vi "Teleop (2).vi"(10 "Match Info":T2={"Autonomous Elapsed Seconds"=0.0, "TeleOp Elapsed Seconds"=0.0, "Disabled Elapsed Seconds"=0.0, "Visited Autonomous"=FALSE, "Visited TeleOp"=FALSE, "Visited Disabled"=FALSE, "Autonomous Settings"={"Autonomous Style"=enum."Independent", "VI Refnum"=refnum}}, 11 "Call Context":T3) -> ()   [LabVIEW 2016]
doc: "This VI is called for each TeleOp packet received from the DS where the robot is not disabled. It is often used to read from the joysticks and update I/O or to update setpoints for timed control loops. It should complete and return within 20 milliseconds or it may miss DS packets."
uses:
  <vilib>/Rock Robotics/WPI/DriverStation/WPI_DriverStationDerivedRobotMode.ctl
  <vilib>/Rock Robotics/WPI/DriverStation/WPI_DriverStationMatch Info.ctl
  <vilib>/Rock Robotics/SystemInterfaces/AI/FPGA_AIGyroChannel.ctl
  <vilib>/Rock Robotics/Network Tables/NT Read Boolean.vi
  <vilib>/Rock Robotics/Network Tables/NT Read Number.vi
  <vilib>/Rock Robotics/WPI/Utilities/WPI_GetSetVariantRefNum.vi
  <vilib>/Rock Robotics/Network Tables/NT Write Boolean.vi
  <vilib>/Rock Robotics/Network Tables/NT Write Number.vi
  <vilib>/Rock Robotics/Network Tables/NT Write Boolean Array.vi
  <vilib>/Rock Robotics/Network Tables/NT Write Numeric Array.vi
  <vilib>/Rock Robotics/WPI/Solenoid/Deprecated/WPI_SolenoidSetBool.vi
  <vilib>/Rock Robotics/WPI/Ultrasonic/WPI_SonarMB1010AnalogRefNum Registry Get.vi
  <vilib>/Rock Robotics/WPI/Ultrasonic/WPI_SonarMB1010AnalogGetRange.vi
  PDP Currents Variable.vi
  <vilib>/Rock Robotics/WPI/Gyro/WPI_GyroAnalogOpen.vi
panel:
  out "gyro":dbl
  out "sonar distance (inches)":dbl
  out "Encoder Loop 2":string
  out "Encoder Loop":dbl
  out "gyro step two":dbl
  out "Encoder Rate":dbl
  out "Encoder State":string
  out "Encoder Direction":string
  out "Distance 2":dbl
  out "Angle 2":dbl
  out "Distance":dbl
  in  "Gain (VoltsPerDegree/Second)":dbl=0.007
  in  "Channel":T1
  in  "Reset Zero Position":bool
  in  "stop":bool
  out "Angle":dbl(knob) scale=0.0..360.0
  out "all currents (A) 2":dbl[](array[numeric])
  out "all currents (A)":dbl[](array[numeric])
  out "Enabled":bool
  out "Compressor Running":bool
  out "Sample Slider 0":dbl(slide) scale=0.0..5.0
  out "Sample Boolean 1":bool
  out "Sample Boolean 0":bool
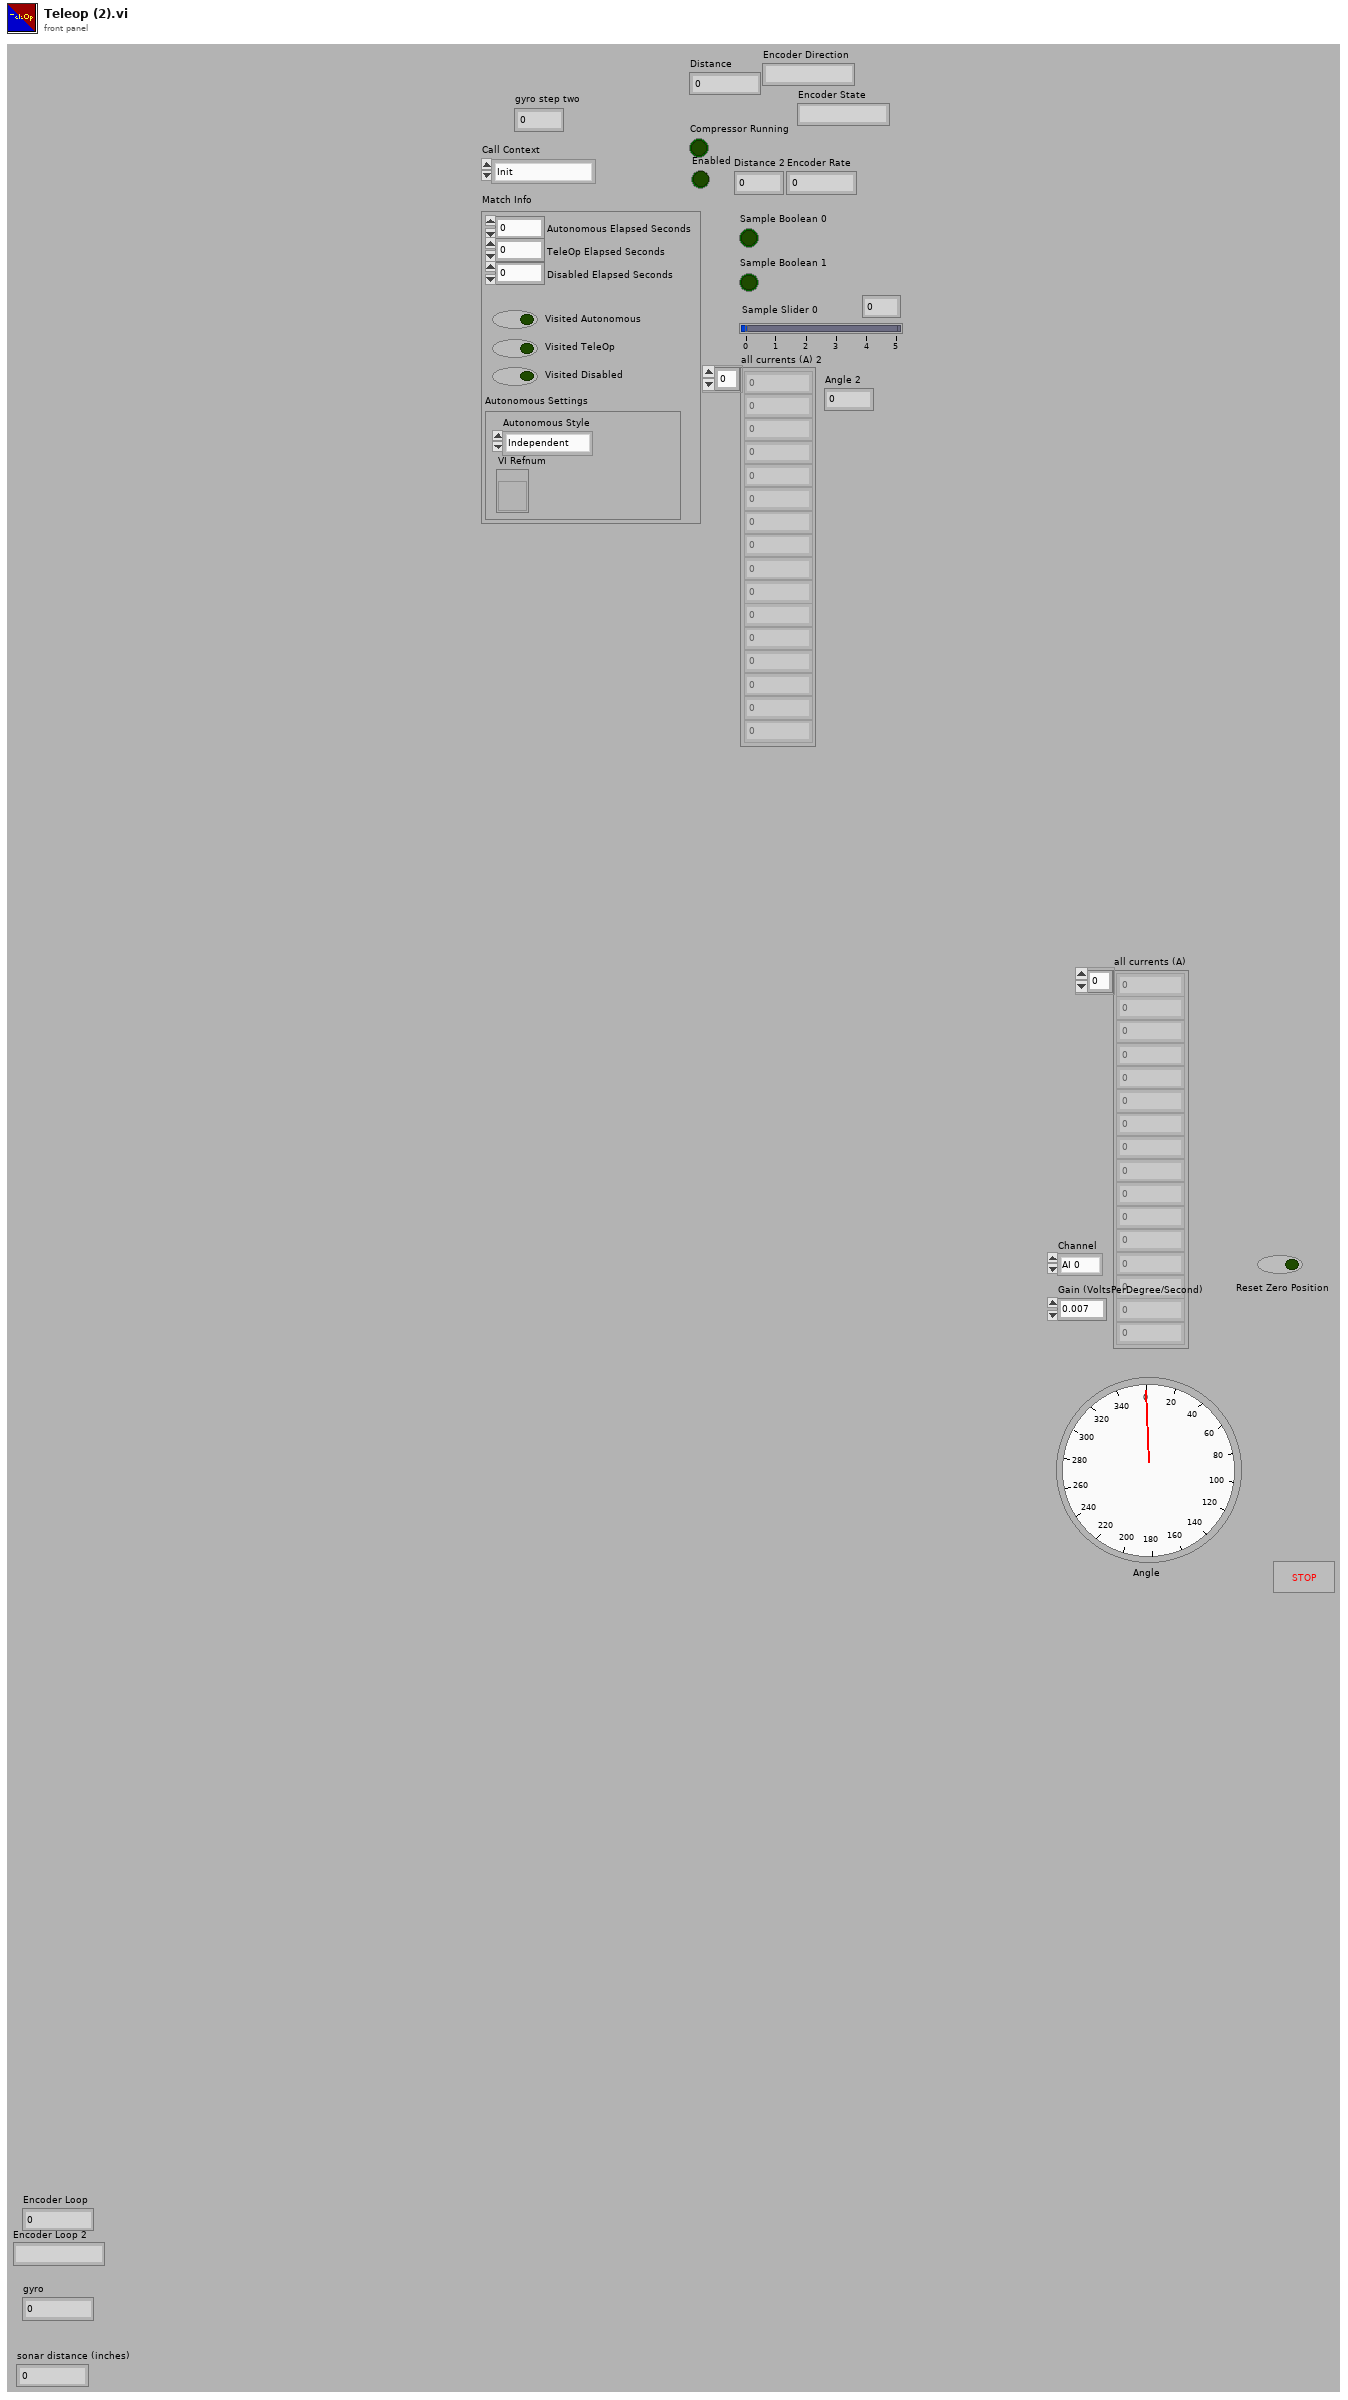
[diagram p1: front panel]
types:
  T1 = typedef "FPGA_AIGyroChannel.ctl" = enum8{"AI 0", "AI 1", "Invalid"}
  T2 = typedef "WPI_DriverStationMatch Info.ctl" = cluster{"Autonomous Elapsed Seconds":dbl, "TeleOp Elapsed Seconds":dbl, "Disabled Elapsed Seconds":dbl, "Visited Autonomous":bool, "Visited TeleOp":bool, "Visited Disabled":bool, "Autonomous Settings":cluster{"Autonomous Style":enum16{"Iterative", "Independent"}, "VI Refnum":refnum<vi>}}
  T3 = typedef "WPI_DriverStationDerivedRobotMode.ctl" = enum16{"Init", "Execute", "Stop"}
  T4 = typedef "WPI_JoystickDevRef.ctl" = cluster{"Device":T5}
  T5 = typedef "WPI_JoystickDeviceEnum.ctl" = enum16{"USB 0", "USB 1", "USB 2", "USB 3", "USB 4", "USB 5"}
  T6 = typedef "WPI_CompressorDevRef.ctl" = cluster{"DevStatus":errorcluster, "Pneumatics Control Module":u8}
  T7 = typedef "WPI_SonarMB1010AnalogDeviceRef.ctl" = cluster{"AIDeviceRef":T8, "Scaling factor (V/in)":dbl, "Average Bits":u8}
  T8 = typedef "WPI_AnalogChannelDevRef.ctl" = cluster{"DevStatus":errorcluster, "Analog Channel":T9}
  T9 = typedef "FPGA_AIChannel.ctl" = enum8{"AI 0", "AI 1", "AI 2", "AI 3", "AI MXP 0", "AI MXP 1", "AI MXP 2", "AI MXP 3", "Invalid"}
  T10 = typedef "WPI_SolenoidDevRef.ctl" = cluster{"DevStatus":errorcluster, "Pneumatics Control Module":u8, "Forward Solenoid Channel":T11, "Reverse Solenoid Channel":T11}
  T11 = typedef "WPI_SolenoidChannel.ctl" = enum8{"Solenoid 0", "Solenoid 1", "Solenoid 2", "Solenoid 3", "Solenoid 4", "Solenoid 5", "Solenoid 6", "Solenoid 7", "Invalid"}
  T12 = typedef "WPI_SwitchDevRef.ctl" = cluster{"DevStatus":errorcluster, "DIO Channel":T13, "CntIndex":T14, "Normally Closed":bool}
  T13 = typedef "FPGA_DIOChannel.ctl" = enum8{"DIO 0", "DIO 1", "DIO 2", "DIO 3", "DIO 4", "DIO 5", "DIO 6", "DIO 7", "DIO 8", "DIO 9", "DIO MXP 0", "DIO MXP 1", "DIO MXP 2", "DIO MXP 3", "DIO MXP 4", "DIO MXP 5", "DIO MXP 6", "DIO MXP 7", "DIO MXP 8", "DIO MXP 9", "DIO MXP 10", "DIO MXP 11", "DIO MXP 12", "DIO MXP 13", "DIO MXP 14", "DIO MXP 15", "SPI Port CS1", "SPI Port CS2", "SPI Port CS3", "SPI Port MISO", "SPI Port MOSI", "Invalid"}
  T14 = typedef "FPGA_CounterCtrSystemIndex.ctl" = enum8{"Ctr 0", "Ctr 1", "Ctr 2", "Ctr 3", "Ctr 4", "Ctr 5", "Ctr 6", "Ctr 7", "Invalid"}
  T15 = typedef "WPI_RobotDriveDevRef.ctl" = cluster{"DevStatus":errorcluster, "Motors[]":T16[], "Square Inputs":bool, "Max Output":dbl}
  T16 = typedef "WPI_MotorControlDeviceRef.ctl" = cluster{"DeviceStatus":errorcluster, "Type":T17, "PWM":cluster{"PWM Channel":T18, "DeadBand":T19}, "CAN":cluster{"Device Number":u8, "SetOutput VI Ref":variant, "GetOutput VI Ref":variant, "Enable VI Ref":variant, "Disable VI Ref":variant, "Data":variant}, "Invert":bool}
  T17 = typedef "WPI_MotorControlType.ctl" = enum16{"PWM", "CAN"}
  T18 = typedef "FPGA_DIOPWMChannel.ctl" = enum8{"PWM 0", "PWM 1", "PWM 2", "PWM 3", "PWM 4", "PWM 5", "PWM 6", "PWM 7", "PWM 8", "PWM 9", "PWM MXP 0", "PWM MXP 1", "PWM MXP 2", "PWM MXP 3", "PWM MXP 4", "PWM MXP 5", "PWM MXP 6", "PWM MXP 7", "PWM MXP 8", "PWM MXP 9", "Invalid"}
  T19 = typedef "WPI_PWMDeadband.ctl" = cluster{"Name":string, "maxPositivePwm":i32, "minPositivePwm":i32, "centerPwm":i32, "maxNegativePwm":i32, "minNegativePwm":i32, "angularRange":u16}
  T20 = typedef "WPI_GyroDevRef.ctl" = cluster{"DevStatus":errorcluster, "Analog Channel":T9, "Offset":dbl, "Gain (VoltsPerDegree/Second)":dbl, "Gyro Type":enum16{"Analog", "XRS450"}, "Handle":i32, "SPI Bus":T21, "Device Found":bool, "Sample Rate":dbl, "Calibrate On Open":bool}
  T21 = typedef "spi_bus.ctl" = enum16{"SPI On-Board, CS0", "SPI On-Board, CS1", "SPI On-Board, CS2", "SPI On-Board, CS3", "SPI MXP", "Invalid"}
  T22 = typedef "WPI_EncoderDevRef.ctl" = cluster{"DevStatus":errorcluster, "EncoderIndex":T23, "CounterIndex":T14, "DistancePerCount":dbl, "Decoding Type":T24}
  T23 = typedef "FPGA_EncoderIdx.ctl" = enum8{"Enc 0", "Enc 1", "Enc 2", "Enc 3", "Enc 4", "Enc 5", "Enc 6", "Enc 7", "Invalid"}
  T24 = typedef "WPI_EncoderType.ctl" = enum16{"1x", "2x", "4x"}
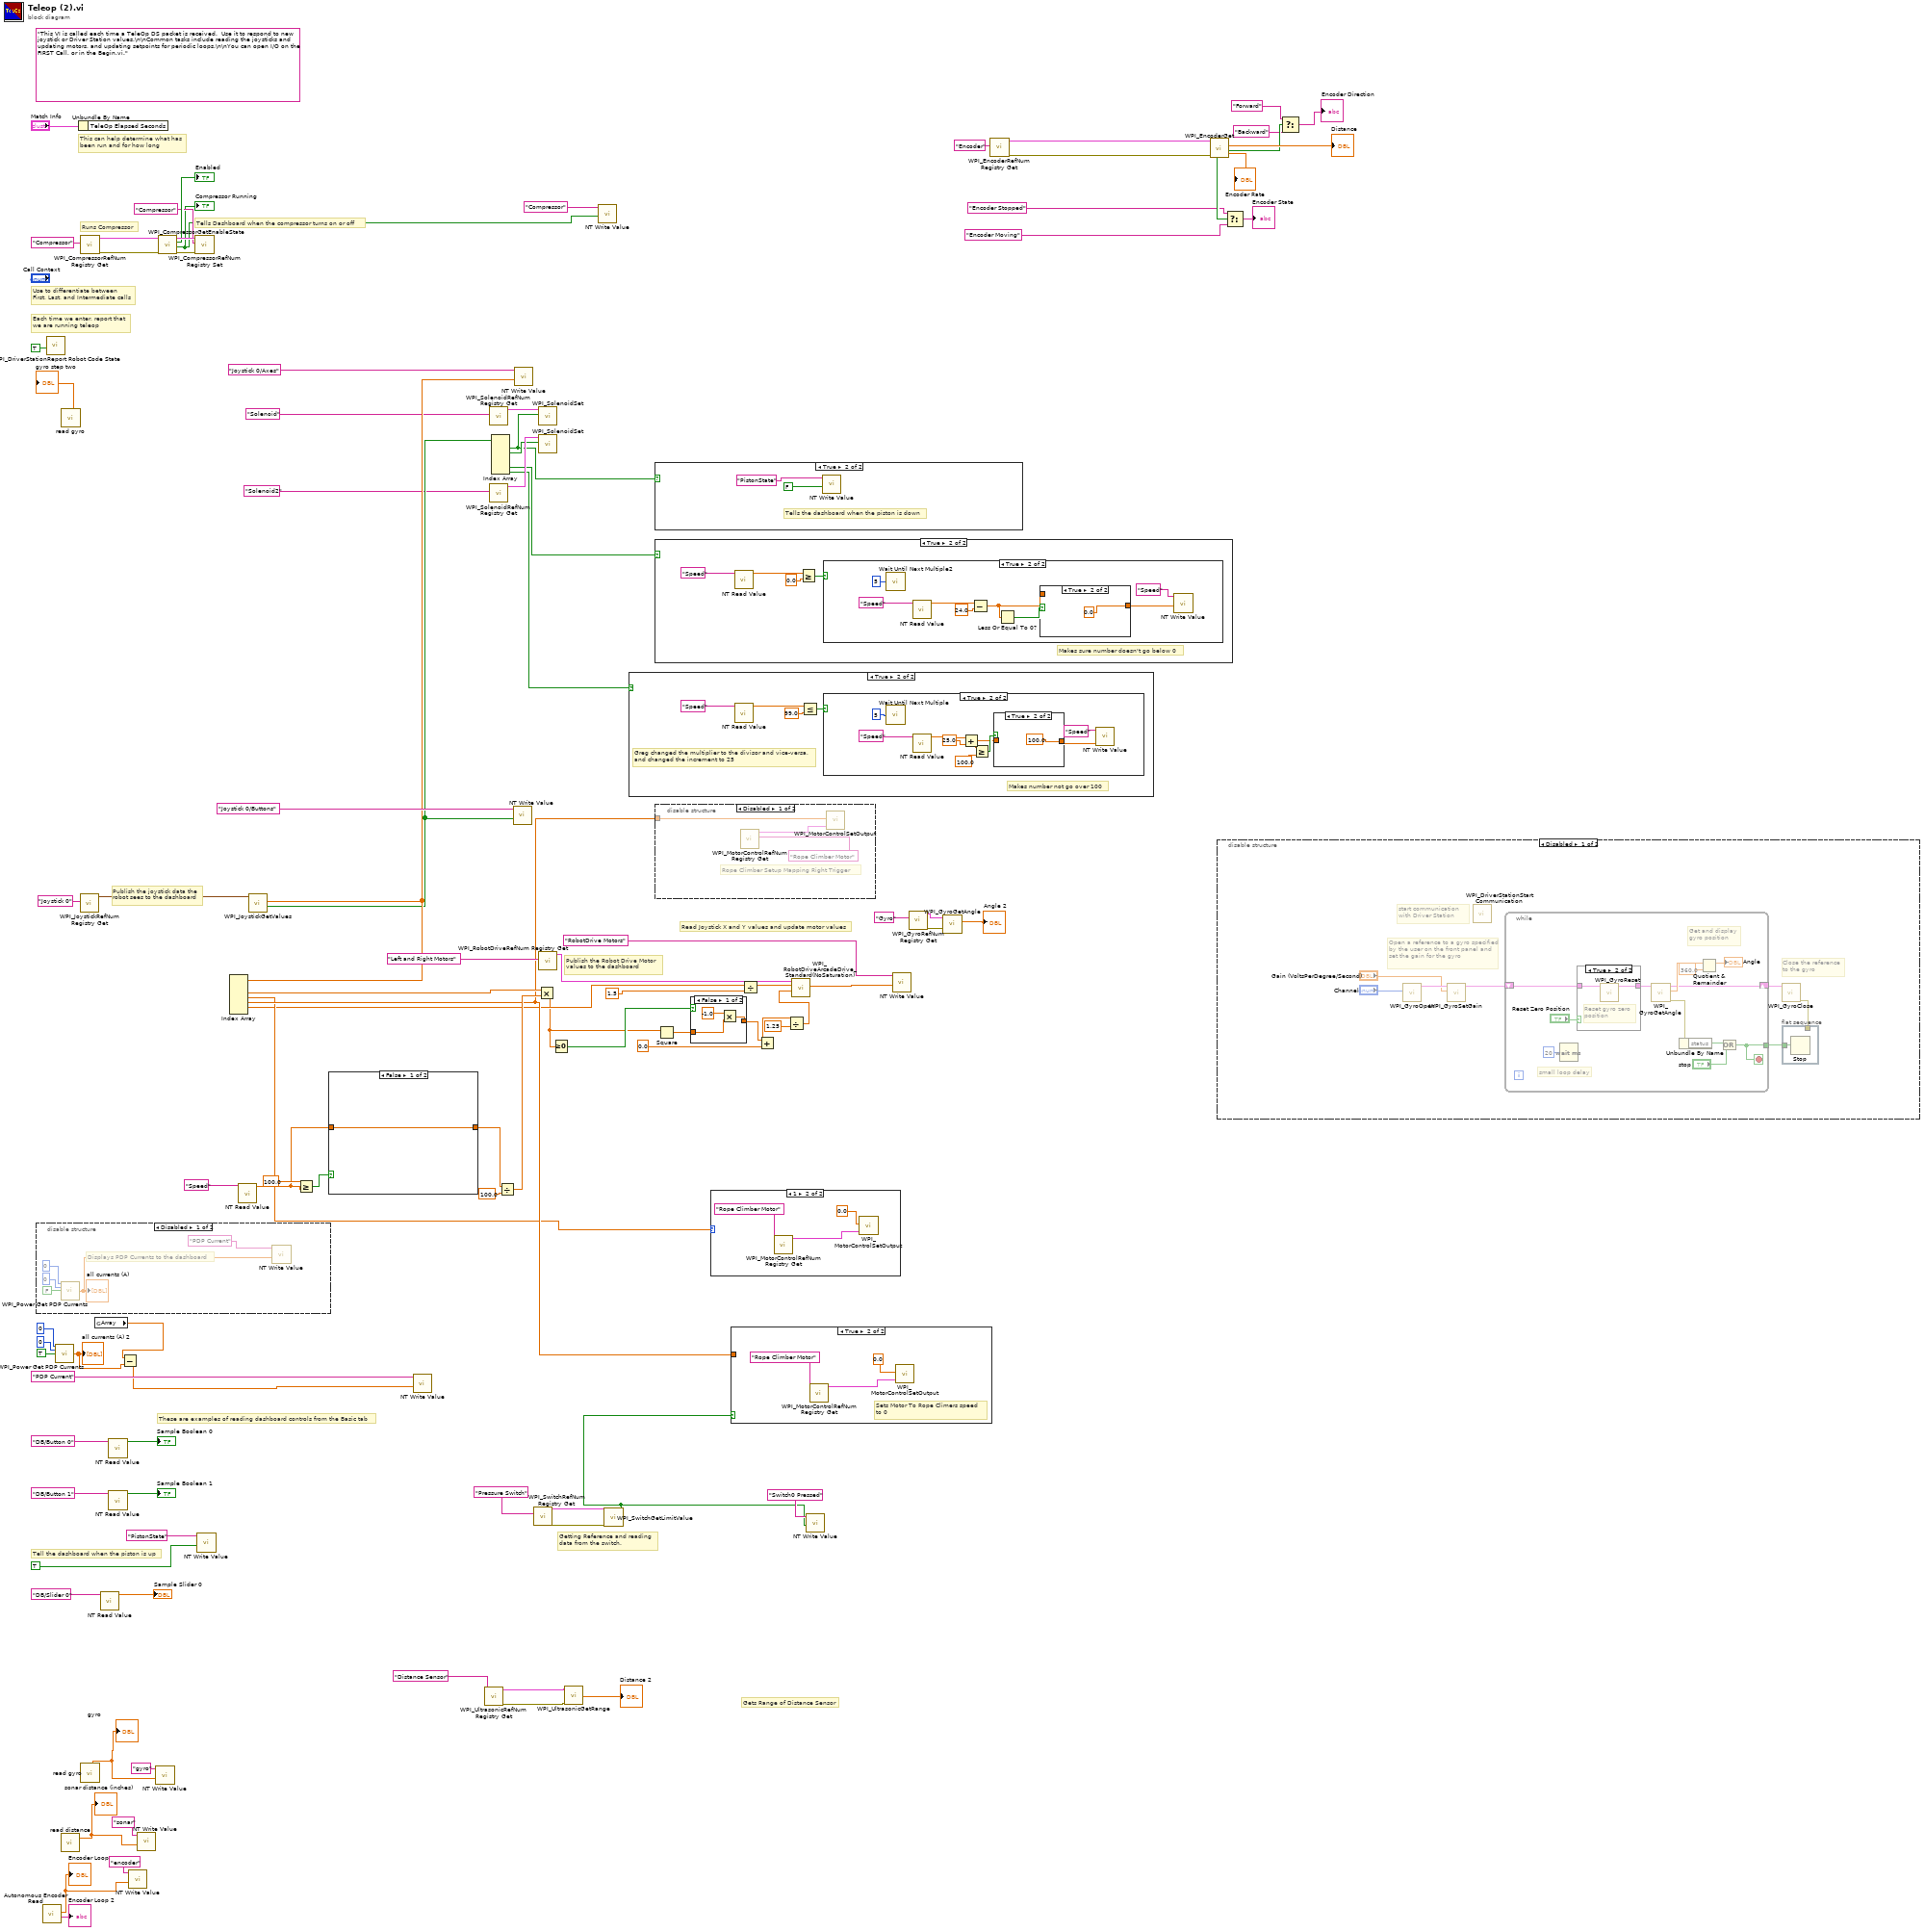
[diagram p0: block diagram]
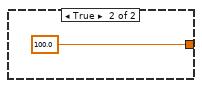
[diagram p3: hidden frame]
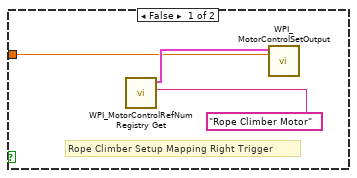
[diagram p8: hidden frame]
diagram:
  (unwired) "This VI is called each time a TeleOp DS packet is received.  Use it to respond to new joystick or Driver Station values.\n\nCommon tasks include reading the joysticks and updating motors, and updating setpoints for periodic loops.\n\nYou can open I/O on the FIRST Call, or in the Begin.vi."
  # "Gets Range of Distance Sensor"
  # "Getting Reference and reading \ndata from the switch."
  # "Tell the dashboard when the piston is up"
  # "Publish the joystick data the\nrobot sees to the dashboard"
  # "Publish the Robot Drive Motor\nvalues to the dashboard"
  # "Read Joystick X and Y values and update motor values"
  # "Tells Dashboard when the compressor turns on or off"
  # "Runs Compressor"
  # "These are examples of reading dashboard controls from the Basic tab"
  # "Each time we enter, report that\nwe are running teleop"
  # "Use to differentiate between\nFirst, Last, and Intermediate calls"
  # "This can help determine what has\nbeen run and for how long"
  n1 = disable-structure shown="Disabled" {
    frame Disabled {
      # "Displays PDP Currents to the dashboard"
      n2 = call <vilib>:"WPI_Power Get PDP Currents.vi"("Power Distribution Panel (0)"=u8 0, "PDP Channel"=0, "Tare Currents?"=FALSE) -> ("all currents (A)"=w102:dbl[])  [unwired: 10 in, 2 out]
      "all currents (A)" <- w102
      n3 = call-poly <vilib>:"NT Write Value.vi"("Numeric Array"=w102, "Name"="PDP Current") -> ()  [unwired: 9 in, 1 out]
    }
    frame Enabled {
    }
  }
  n4 = call "Autonomous Encoder Read.vi"() -> ("Encoder Direction"=→"Encoder Loop 2":string, "Encoder Distance"=w2:dbl)  [unwired: 9 in, 1 out]
  "Encoder Loop" <- w2
  n5 = call <vilib>:"WPI_DriverStationReport Robot Code State.vi"("TeleOp"=TRUE ("Autonomous")) -> ()  [unwired: 10 in, 1 out]
  n6 = call <vilib>:"WPI_Power Get PDP Currents.vi"("Power Distribution Panel (0)"=u8 0, "PDP Channel"=0, "Tare Currents?"=TRUE) -> ("all currents (A)"=w54:dbl[])  [unwired: 10 in, 2 out]
  "all currents (A) 2" <- w54
  n7 = call "read distance.vi"() -> ("Distance 2"=w5:dbl)  [unwired: 10 in, 1 out]
  "sonar distance (inches)" <- w5
  n8 = call "read gyro.vi"() -> ("Angle 2"=→"gyro step two":dbl)  [unwired: 10 in, 1 out]
  n9 = Unbundle By Name("Match Info") -> ()  [unwired: 1 out]
  n10 = call <vilib>:"WPI_JoystickRefNum Registry Get.vi"("refnum name"="Joystick 0") -> ("JoystickDevRef"=w79:T4)  [unwired: 1 in, 9 out]
  n11 = call <vilib>:"WPI_CompressorRefNum Registry Get.vi"("refnum name"="Compressor") -> ("error out"=w89:errorcluster, "CompressorDevRef"=w91:T6)  [unwired: 9 in]
  n12 = call "read gyro.vi"() -> ("Angle 2"=w7:dbl)  [unwired: 10 in, 1 out]
  "gyro" <- w7
  n13 = global read "PDP Currents Variable.vi" "Array"() -> (w52:dbl[])
  n14 = call-poly <vilib>:"NT Read Value.vi"("Name"="DB/Slider 0" ("refnum name")) -> ("Numeric"=→"Sample Slider 0":dbl)  [unwired: 9 in, 1 out]
  n15 = call-poly <vilib>:"NT Read Value.vi"("Name"="DB/Button 0" ("refnum name")) -> ("Boolean"=→"Sample Boolean 0":bool)  [unwired: 9 in, 1 out]
  n16 = call-poly <vilib>:"NT Read Value.vi"("Name"="DB/Button 1" ("refnum name")) -> ("Boolean"=→"Sample Boolean 1":bool)  [unwired: 9 in, 1 out]
  n17 = Subtract(x=w52, y=w54) -> (x-y=w53:dbl[])
  n18 = call-poly <vilib>:"NT Write Value.vi"("Numeric"=w2, "Name"="encoder") -> ()  [unwired: 9 in, 1 out]
  n19 = call-poly <vilib>:"NT Write Value.vi"("Numeric"=w5, "Name"="sonar") -> ()  [unwired: 9 in, 1 out]
  n20 = call-poly <vilib>:"NT Write Value.vi"("Numeric"=w7, "Name"="gyro") -> ()  [unwired: 9 in, 1 out]
  n21 = call <vilib>:"WPI_CompressorGetEnableState.vi"("error in (no error)"=w89, "CompressorDevRef"=w91) -> ("error out"=w88:errorcluster, "Compressor Running"=w83:bool, "Enabled"=→"Enabled":bool, "CompressorDevRef"=w90:T6)  [unwired: 6 in]
  "Compressor Running" <- w83
  n22 = call <vilib>:"WPI_CompressorRefNum Registry Set.vi"("error in (no error)"=w88, "refnum name"="Compressor", "CompressorDevRef"=w90) -> ()  [unwired: 7 in, 2 out]
  n23 = call-poly <vilib>:"NT Write Value.vi"("Boolean"=TRUE, "Name"="PistonState") -> ()  [unwired: 9 in, 1 out]
  n24 = call-poly <vilib>:"NT Read Value.vi"("Name"="Speed") -> ("Numeric"=w16:dbl)  [unwired: 9 in, 1 out]
  n25 = call <vilib>:"WPI_JoystickGetValues.vi"("JoystickDevRef"=w79) -> ("Buttons"=w73:bool[], "Axes"=w76:dbl[])  [unwired: 6 in, 3 out]
  n26 = Index Array(array=w76) -> (element #2=w64:dbl, element #3=w45:dbl, element #4=w46:dbl, element #5=w20:dbl)  [unwired: 6 in, 2 out]
  n27 = Greater Or Equal?(x=100.0, y=w16) -> (x >= y?=w18:bool)
  n28 = case shown="False" w18 {
    tunnel: [w105 100.0 ("Numeric")] -> w17
    tunnel: w16 -> [w105 _]
    frame False {
    }
    frame True {
    }
  }
  n29 = call-poly <vilib>:"NT Write Value.vi"("Numeric Array"=w53, "Name"="PDP Current") -> ()  [unwired: 9 in, 1 out]
  n30 = call-poly <vilib>:"WPI_UltrasonicRefNum Registry Get.vi"("refnum name"="Distance Sensor") -> ("error out"=w31:errorcluster, "SonarMB1010AnalogDevRef"=w33:T7)  [unwired: 9 in]
  n31 = call <vilib>:"WPI_SolenoidRefNum Registry Get.vi"("refnum name"="Solenoid") -> ("SolenoidDevRef"=w69:T10)  [unwired: 9 in, 1 out]
  n32 = call <vilib>:"WPI_SolenoidRefNum Registry Get.vi"("refnum name"="Solenoid2") -> ("SolenoidDevRef"=w71:T10)  [unwired: 9 in, 1 out]
  n33 = Index Array(array=w73) -> (element #1=w67:bool, element #2=w68:bool, element #5=w59:bool, element #6=w60:bool)  [unwired: 6 in, 2 out]
  n34 = Divide(x=w17, y=100.0 ("x")) -> (x/y=w61:dbl)
  n35 = call-poly <vilib>:"NT Write Value.vi"("Boolean Array"=w73, "Name"="Joystick 0/Buttons") -> ()  [unwired: 9 in, 1 out]
  n36 = call-poly <vilib>:"NT Write Value.vi"("Numeric Array"=w76, "Name"="Joystick 0/Axes") -> ()  [unwired: 9 in, 1 out]
  n37 = call <vilib>:"WPI_SwitchRefNum Registry Get.vi"("refnum name"="Pressure Switch") -> ("error out"=w49:errorcluster, "SwitchDevRef"=w50:T12)  [unwired: 9 in]
  n38 = Multiply(x=w64, y=w61) -> (x*y=w10:dbl)
  n39 = call-poly <vilib>:"WPI_SolenoidSet.vi"("Value"=w67, "SolenoidDevRef"=w69) -> ()  [unwired: 8 in, 2 out]
  n40 = call-poly <vilib>:"WPI_SolenoidSet.vi"("Value"=w68, "SolenoidDevRef"=w71) -> ()  [unwired: 8 in, 2 out]
  n41 = call <vilib>:"WPI_RobotDriveRefNum Registry Get.vi"("refnum name"="Left and Right Motors") -> ("RobotDriveDevRef"=w81:T15)  [unwired: 1 in, 9 out]
  n42 = Greater Or Equal To 0?(x=w10) -> (x >= 0?=w11:bool)
  n43 = call-poly <vilib>:"WPI_UltrasonicGetRange.vi"("error in"=w31, "SonarMB1010AnalogDevRef"=w33) -> ("Distance"=→"Distance 2":dbl)  [unwired: 7 in, 2 out]
  n44 = call-poly <vilib>:"NT Write Value.vi"("Boolean"=w83, "Name"="Compressor") -> ()  [unwired: 9 in, 1 out]
  n45 = call <vilib>:"WPI_SwitchGetLimitValue.vi"("error in (no error)"=w49, "SwitchDevRef"=w50) -> ("Switch Pressed"=w47:bool)  [unwired: 7 in, 2 out]
  n46 = case shown="True" w60 {
    frame False {
    }
    frame True {
      # "Makes number not go over 100"
      # "Greg changed the multiplier to the divisor and vice-versa,\nand changed the increment to 25"
      n47 = call-poly <vilib>:"NT Read Value.vi"("Name"="Speed") -> ("Numeric"=w108:dbl)  [unwired: 9 in, 1 out]
      n48 = Less Or Equal?(x=w108, y=99.0) -> (x <= y?=w109:bool)
      n49 = case shown="True" w109 {
        frame False {
        }
        frame True {
          n50 = call "Wait Until Next Multiple"("Count(mSec)"=u32 5) -> ()  [unwired: 1 out]
          n51 = call-poly <vilib>:"NT Read Value.vi"("Name"="Speed") -> ("Numeric"=w116:dbl)  [unwired: 9 in, 1 out]
          n52 = Add(x=w116, y=25.0) -> (x+y=w111:dbl)
          n53 = Greater Or Equal?(x=w111, y=100.0) -> (x >= y?=w113:bool)
          n54 = case shown="True" w113 {
            tunnel: [w120 100.0 ("Numeric")] -> w114
            tunnel: w111 -> [w120 _]
            frame False {
            }
            frame True {
            }
          }
          n55 = call-poly <vilib>:"NT Write Value.vi"("Numeric"=w114, "Name"="Speed") -> ()  [unwired: 9 in, 1 out]
        }
      }
    }
  }
  n56 = case shown="True" w67 {
    frame False {
    }
    frame True {
      # "Tells the dashboard when the piston is down"
      n57 = call-poly <vilib>:"NT Write Value.vi"("Boolean"=FALSE, "Name"="PistonState") -> ()  [unwired: 9 in, 1 out]
    }
  }
  n58 = case shown="True" w59 {
    frame False {
    }
    frame True {
      # "Makes sure number doesn't go below 0"
      n59 = call-poly <vilib>:"NT Read Value.vi"("Name"="Speed") -> ("Numeric"=w126:dbl)  [unwired: 9 in, 1 out]
      n60 = Greater Or Equal?(x=w126, y=0.0) -> (x >= y?=w124:bool)
      n61 = case shown="True" w124 {
        frame False {
        }
        frame True {
          n62 = call "Wait Until Next Multiple2"("Count(mSec)"=u32 5) -> ()  [unwired: 1 out]
          n63 = call-poly <vilib>:"NT Read Value.vi"("Name"="Speed") -> ("Numeric"=w134:dbl)  [unwired: 9 in, 1 out]
          n64 = Subtract(x=w134, y=24.0) -> (x-y=w128:dbl)
          n65 = Less Or Equal To 0?(x=w128) -> (x <= 0?=w130:bool)
          n66 = case shown="True" w130 {
            tunnel: [w136 0.0 ("Numeric")] -> w129
            tunnel: w128 -> [w136 _]
            frame False {
            }
            frame True {
            }
          }
          n67 = call-poly <vilib>:"NT Write Value.vi"("Numeric"=w129, "Name"="Speed") -> ()  [unwired: 9 in, 1 out]
        }
      }
    }
  }
  n68 = disable-structure shown="Disabled" {
    disable-tunnel: w46 -> [w138 _]
    frame Disabled {
      # "Rope Climber Setup Mapping Right Trigger"
      n69 = call <vilib>:"WPI_MotorControlRefNum Registry Get.vi"("refnum name"="Rope Climber Motor") -> ("MotorControlDevRef"=w139:T16)  [unwired: 9 in, 1 out]
      n70 = call <vilib>:"WPI_MotorControlSetOutput.vi"("Output"=w138, "MotorControlDevRef"=w139) -> ()  [unwired: 7 in, 3 out]
    }
    frame Enabled {
    }
  }
  n71 = Square(x=w10) -> (x^2=w9:dbl)
  n72 = case shown="False" w11 {
    tunnel: w9 -> [w143 w144]
    tunnel: [w141 w144] -> w8
    frame False {
      n73 = Multiply(x=-1.0, y=w143) -> (x*y=w141:dbl)
    }
    frame True {
    }
  }
  n74 = case shown="1" w45 {
    frame 0, Default {
    }
    frame 1 {
      n75 = call <vilib>:"WPI_MotorControlRefNum Registry Get.vi"("refnum name"="Rope Climber Motor") -> ("MotorControlDevRef"=w147:T16)  [unwired: 9 in, 1 out]
      n76 = call <vilib>:"WPI_MotorControlSetOutput.vi"("Output"=0.0 ("Motor Output"), "MotorControlDevRef"=w147) -> ()  [unwired: 7 in, 3 out]
    }
  }
  n77 = case shown="True" w47 {
    tunnel: w46 -> [w148 _]
    frame False {
      # "Rope Climber Setup Mapping Right Trigger"
      n78 = call <vilib>:"WPI_MotorControlRefNum Registry Get.vi"("refnum name"="Rope Climber Motor") -> ("MotorControlDevRef"=w149:T16)  [unwired: 9 in, 1 out]
      n79 = call <vilib>:"WPI_MotorControlSetOutput.vi"("Output"=w148, "MotorControlDevRef"=w149) -> ()  [unwired: 7 in, 3 out]
    }
    frame True {
      # "Sets Motor To Rope Climers speed \nto 0"
      n80 = call <vilib>:"WPI_MotorControlRefNum Registry Get.vi"("refnum name"="Rope Climber Motor") -> ("MotorControlDevRef"=w153:T16)  [unwired: 9 in, 1 out]
      n81 = call <vilib>:"WPI_MotorControlSetOutput.vi"("Output"=0.0 ("Motor Output"), "MotorControlDevRef"=w153) -> ()  [unwired: 7 in, 3 out]
    }
  }
  n82 = Divide(x=w20, y=1.5) -> (x/y=w43:dbl)
  n83 = Add(x=w8, y=0.0) -> (x+y=w13:dbl)
  n84 = Divide(x=w13, y=1.25) -> (x/y=w12:dbl)
  n85 = call <vilib>:"WPI_RobotDriveArcadeDrive_Standard(NoSaturation).vi"("Y axis value"=w12, "X axis value"=w43, "RobotDriveDevRef"=w81) -> ("Motor Values"=w75:dbl[])  [unwired: 1 in, 7 out]
  n86 = call-poly <vilib>:"NT Write Value.vi"("Boolean"=w47, "Name"="Switch0 Pressed") -> ()  [unwired: 9 in, 1 out]
  n87 = call-poly <vilib>:"NT Write Value.vi"("Numeric Array"=w75, "Name"="RobotDrive Motors") -> ()  [unwired: 9 in, 1 out]
  n88 = call <vilib>:"WPI_GyroRefNum Registry Get.vi"("refnum name"="Gyro") -> ("error out"=w35:errorcluster, "GyroDevRef"=w36:T20)  [unwired: 9 in]
  n89 = call <vilib>:"WPI_GyroGetAngle.vi"("error in"=w35, "GyroDevRef"=w36) -> ("Angle"=→"Angle 2":dbl)  [unwired: 5 in, 4 out]
  n90 = call <vilib>:"WPI_EncoderRefNum Registry Get.vi"("refnum name"="Encoder") -> ("error out"=w40:errorcluster, "EncoderDevRef"=w41:T22)  [unwired: 9 in]
  n91 = call <vilib>:"WPI_EncoderGet.vi"("error in (no error)"=w40, "EncoderDevRef"=w41) -> ("Direction"=w30:bool, "Distance"=→"Distance":dbl, "Rate"=→"Encoder Rate":dbl, "Stopped"=w26:bool)  [unwired: 4 in, 2 out]
  n92 = disable-structure shown="Disabled" {
    frame Disabled {
      # "start communication with Driver Station"
      # "Close the reference\nto the gyro"
      # "Open a reference to a gyro specified by the user on the front panel and set the gain for the gyro"
      n93 = call-poly <vilib>:"WPI_GyroOpen.vi"("Analog Channel"="Channel") -> ("GyroDevRef"=w159:T20)  [unwired: 8 in, 2 out]
      n94 = call <vilib>:"WPI_GyroSetGain.vi"("Gain (VoltsPerDegree/Second)"="Gain (VoltsPerDegree/Second)", "GyroDevRef"=w159) -> ("GyroDevRef"=w158:T20)  [unwired: 1 in, 8 out]
      n95 = call <vilib>:"WPI_DriverStationStart Communication.vi"() -> ()  [unwired: 2 in, 10 out]
      n96 = while {
        shift-right: [w169] -> w160
        shift-left: w158 -> [w172]
        tunnel: [w167] -> w155
        stop <- w167 stop-if-true
        # "small loop delay"
        # "Get and display\ngyro position"
        n97 = Wait (ms)(milliseconds to wait=u32 20) -> ()  [unwired: 1 out]
        n98 = case shown="True" "Reset Zero Position" {
          tunnel: w172 -> [w174 w176]
          tunnel: [w174 w175] -> w171
          frame False {
          }
          frame True {
            # "Reset gyro zero \nposition"
            n99 = call <vilib>:"WPI_GyroReset.vi"("GyroDevRef"=w176) -> ("GyroDevRef"=w175:T20)  [unwired: 10 out]
          }
        }
        n100 = call <vilib>:"WPI_GyroGetAngle.vi"("GyroDevRef"=w171) -> ("error out"=w164:errorcluster, "Angle"=w170:dbl, "GyroDevRef"=w169:T20)  [unwired: 1 in, 7 out]
        n101 = Unbundle By Name(w164) -> ("status"=w168:bool)
        n102 = Quotient & Remainder(x=w170, y=360.0) -> (x-y*floor(x/y)=→"Angle":dbl)  [unwired: 1 out]
        n103 = Or(x=w168, y="stop") -> (x .or. y?=w167:bool)
      }
      n104 = call <vilib>:"WPI_GyroClose.vi"("GyroDevRef"=w160) -> ("error out"=w154:errorcluster)  [unwired: 1 in, 9 out]
      n105 = flat-sequence {
        tunnel: w155 -> [w161]
        tunnel: w154 -> [_]
        frame #0 {
          n106 = Stop(stop? (T)=w161) -> ()
        }
      }
    }
    frame Enabled {
    }
  }
  n107 = Select(t="Encoder Stopped", s=w26, f="Encoder Moving") -> (s? t:f=→"Encoder State":string)
  n108 = Select(t="Forward", s=w30, f="Backward") -> (s? t:f=→"Encoder Direction":string)
